vi "PlotColor.vi"(9 "White Palette":bool, 10 "InputColorCode":u8, 11 "Color":T1) -> (3 "Color":u32(colorbox))   [LabVIEW 2020]
uses:
  ColorSelection.ctl
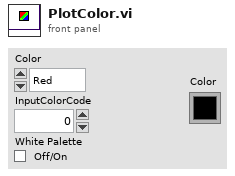
[diagram p1: front panel]
types:
  T1 = typedef "ColorSelection.ctl" = enum16{"Red", "Green", "Blue", "Yellow", "Magenta", "Cyan", "White", "Black"}
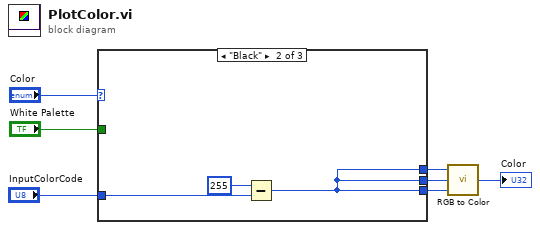
[diagram p0: block diagram]
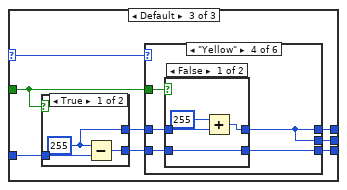
[diagram p3: hidden frame]
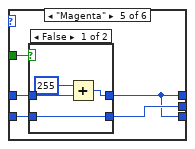
[diagram p8: hidden frame]
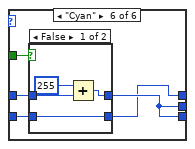
[diagram p10: hidden frame]
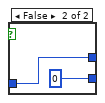
[diagram p12: hidden frame]
diagram:
  n1 = case shown="\"Black\"" "Color" {
    selector: "Color" -> [_ _ w12]
    tunnel: "InputColorCode" -> [w8 w10 w17]
    tunnel: [w8 w9 w16] -> w5
    tunnel: [w8 w9 w15] -> w4
    tunnel: [w8 w9 w14] -> w3
    tunnel: "White Palette" -> [_ _ w13]
    frame "White" {
    }
    frame "Black" {
      n2 = Subtract(x=u8 255, y=w10) -> (x-y=w9:u8)
    }
    frame Default {
      n3 = case shown="True" w13 {
        tunnel: [w59 w63] -> w19
        tunnel: [w61 u8 0] -> w18
        tunnel: w17 -> [w60 w63]
        frame True {
          w59 = u8 255
          n4 = Subtract(x=w59, y=w60) -> (x-y=w61:u8)
        }
        frame False {
        }
      }
      n5 = case shown="\"Yellow\"" w12 {
        tunnel: w19 -> [w21 w23 w25 w29 w40 w51]
        tunnel: w18 -> [w20 w22 w24 w26 w39 w50]
        tunnel: [w21 w22 w24 w27 w37 w48] -> w16
        tunnel: [w20 w23 w24 w27 w38 w49] -> w15
        tunnel: [w20 w22 w25 w28 w37 w49] -> w14
        tunnel: w13 -> [_ _ _ w30 w41 w52]
        frame "Red", Default {
        }
        frame "Green" {
        }
        frame "Blue" {
        }
        frame "Yellow" {
          n6 = case shown="False" w30 {
            tunnel: w29 -> [w34 w36]
            tunnel: [w31 w35] -> w28
            tunnel: [w32 w36] -> w27
            tunnel: w26 -> [w31 w35]
            frame False {
              n7 = Add(x=u8 255, y=w34) -> (x+y=w32:u8)
            }
            frame True {
            }
          }
        }
        frame "Magenta" {
          n8 = case shown="False" w41 {
            tunnel: w40 -> [w45 w47]
            tunnel: [w42 w46] -> w38
            tunnel: [w43 w47] -> w37
            tunnel: w39 -> [w42 w46]
            frame False {
              n9 = Add(x=u8 255, y=w45) -> (x+y=w43:u8)
            }
            frame True {
            }
          }
        }
        frame "Cyan" {
          n10 = case shown="False" w52 {
            tunnel: w51 -> [w56 w58]
            tunnel: [w53 w57] -> w48
            tunnel: [w54 w58] -> w49
            tunnel: w50 -> [w53 w57]
            frame False {
              n11 = Add(x=u8 255, y=w56) -> (x+y=w54:u8)
            }
            frame True {
            }
          }
        }
      }
    }
  }
  n12 = call <vilib>:"RGB to Color.vi"("B"=w3, "G"=w4, "R"=w5) -> ("Color"=→"Color":u32)
